vi "Configure Sweep (Noise).vi"(0 "VISA resource name":refnum<visa-resource-name>, 1 "Stop (10E6 Hz)":dbl=10000000.0 format="%^#_9g", 5 "Measurement Type (6: Phase Noise)":u16(ring)=6 items=["AM Noise"=1, "Baseband Noise"=2, "Phase Noise"=6], 9 "Start (1E3 Hz)":dbl=1000.0 format="%^#_9g", 11 "error in (no error)":errorcluster) -> (4 "VISA resource name out":refnum<visa-resource-name>, 15 "error out":errorcluster)   [LabVIEW 2011, in "Agilent E5052X.lvlib"]
doc: "Sets the range in which measurements will be taken for the any noise measurement including Phase, AM and Baseband Noise.\n\n<b>Note:</b>\n\n1) \"Configure Measurement Characteristics\" VI for Phase, AM or Baseband Noise must be run before this VI."
uses:
  Agilent E5052X.lvlib
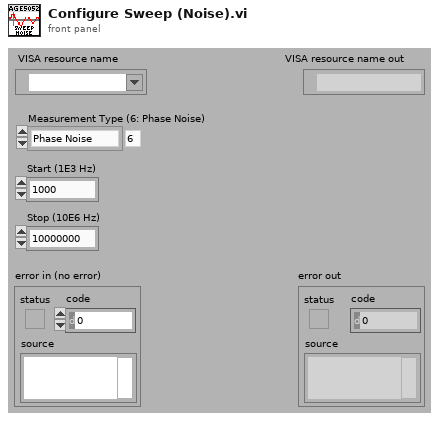
[diagram p1: front panel]
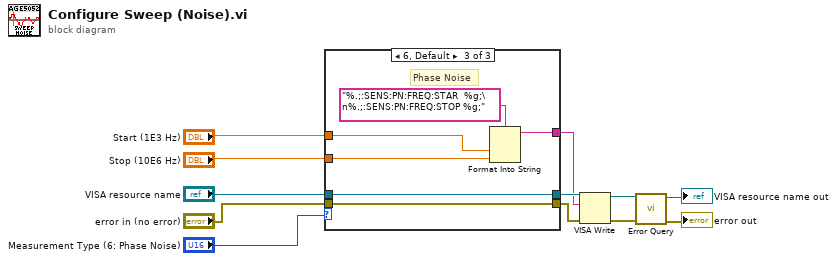
[diagram p0: block diagram]
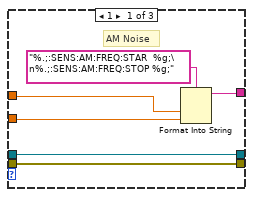
[diagram p2: hidden frame]
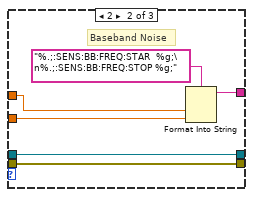
[diagram p3: hidden frame]
diagram:
  n1 = case shown="6, Default" "Measurement Type (6: Phase Noise)" {
    tunnel: "Start (1E3 Hz)" -> [w17 w23 w29]
    tunnel: "Stop (10E6 Hz)" -> [w16 w22 w28]
    tunnel: [w15 w21 w27] -> w8
    tunnel: "VISA resource name" -> [w14 w20 w26]
    tunnel: [w14 w20 w26] -> w10
    tunnel: "error in (no error)" -> [w13 w19 w25]
    tunnel: [w13 w19 w25] -> w9
    frame 1 {
      # "AM Noise"
      n2 = Format Into String(format string="%.;:SENS:AM:FREQ:STAR  %g;\n%.;:SENS:AM:FREQ:STOP %g;", w17, w16) -> (resulting string=w15:string)  [unwired: 2 in, 1 out]
    }
    frame 2 {
      # "Baseband Noise"
      n3 = Format Into String(format string="%.;:SENS:BB:FREQ:STAR  %g;\n%.;:SENS:BB:FREQ:STOP %g;", w23, w22) -> (resulting string=w21:string)  [unwired: 2 in, 1 out]
    }
    frame 6, Default {
      # "Phase Noise"
      n4 = Format Into String(format string="%.;:SENS:PN:FREQ:STAR  %g;\n%.;:SENS:PN:FREQ:STOP %g;", w29, w28) -> (resulting string=w27:string)  [unwired: 2 in, 1 out]
    }
  }
  n5 = VISA Write(VISA resource name=w10, write buffer=w8, error in (no error)=w9) -> (VISA resource name out=w7:refnum<visa-resource-name>, error out=w6:errorcluster)  [unwired: 1 out]
  n6 = call "Error Query.vi"("error in (no error)"=w6, "VISA resource name"=w7) -> ("error out"=→"error out":errorcluster, "VISA resource name out"=→"VISA resource name out":refnum<visa-resource-name>)  [unwired: 6 in, 2 out]
